vi "Configure Sweep (Step).vi"(0 "VISA resource name":refnum<visa-resource-name>, 1 "Step Spacing (0: Linear)":u16(ring) items=["Linear", "Logarithmic"], 2 "Number Of Points (2)":i32=2, 5 "Step Dwell (2 ms)":dbl=0.002, 7 "Frequency Start (100 kHz)":dbl=100000.0, 9 "Frequency Stop (100 kHz)":dbl=100000.0, 11 "error in (no error)":errorcluster, 12 "Power Start (-130 dB)":dbl=-130.0, 13 "Power Stop (-130 dB)":dbl=-130.0) -> (4 "VISA resource name out":refnum<visa-resource-name>, 15 "error out":errorcluster)   [LabVIEW 2009, in "Agilent PSG MXG Series.lvlib"]
doc: "Configures number of points, dwell time, start frequency, stop frequency, start amplitude and stop amplitude in the step sweep mode."
uses:
  Agilent PSG MXG Series.lvlib
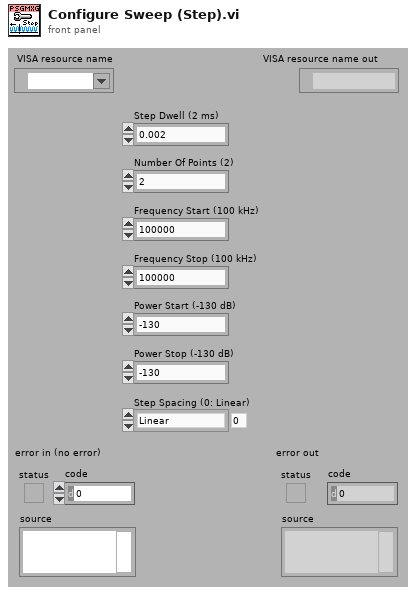
[diagram p1: front panel]
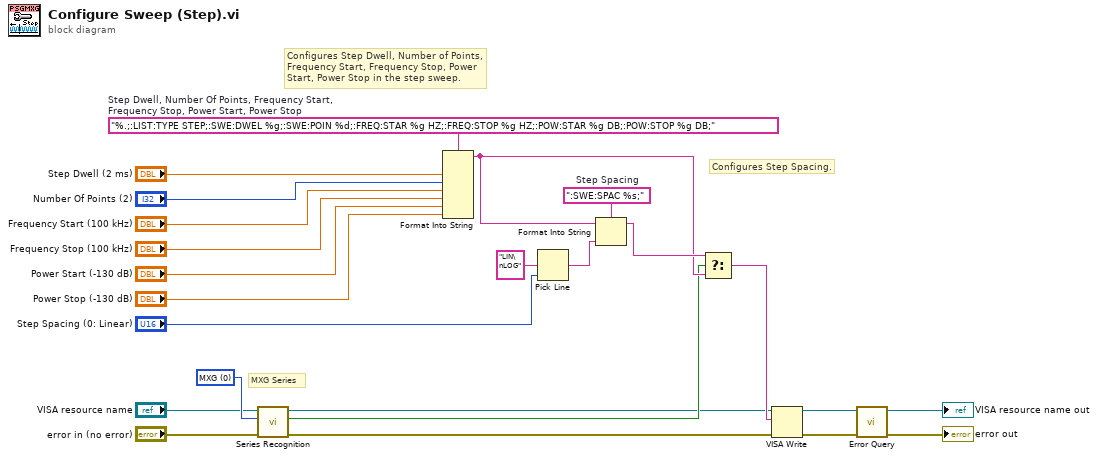
[diagram p0: block diagram]
diagram:
  w5 = u16 0 items=["MXG", "PSG", "PSG-A", "PSG-C", "PSG-D"] ("Series Type (0: MXG)")
  w17 = ":SWE:SPAC %s;"  # Step Spacing
  w24 = "%.;:LIST:TYPE STEP;:SWE:DWEL %g;:SWE:POIN %d;:FREQ:STAR %g HZ;:FREQ:STOP %g HZ;:POW:STAR %g DB;:POW:STOP %g DB;"  # Step Dwell, Number Of Points, Frequency Start, Frequency Stop, Power Start, Power Stop
  # "MXG Series"
  # "Configures Step Spacing."
  # "Configures Step Dwell, Number of Points,\nFrequency Start, Frequency Stop, Power\nStart, Power Stop in the step sweep."
  n1 = call "Series Recognition.vi"("error in (no error)"="error in (no error)", "Series Type (0: MXG)"=w5, "VISA resource name"="VISA resource name") -> ("error out"=w6:errorcluster, "Is Series Correct"=w8:bool, "VISA resource name out"=w7:refnum<visa-resource-name>)  [unwired: 1 in, 5 out]
  n2 = Format Into String(format string=w24, "Step Dwell (2 ms)", "Number Of Points (2)", "Frequency Start (100 kHz)", "Frequency Stop (100 kHz)", "Power Start (-130 dB)", "Power Stop (-130 dB)") -> (resulting string=w12:string)  [unwired: 2 in, 1 out]
  n3 = Pick Line(multi-line string="LIN\nLOG", line index="Step Spacing (0: Linear)") -> (output string=w16:string)  [unwired: 1 out]
  n4 = Format Into String(format string=w17, initial string=w12, w16) -> (resulting string=w13:string)  [unwired: 1 in, 1 out]
  n5 = Select(t=w13, s=w8, f=w12) -> (s? t:f=w11:string)
  n6 = VISA Write(VISA resource name=w7, write buffer=w11, error in (no error)=w6) -> (VISA resource name out=w10:refnum<visa-resource-name>, error out=w9:errorcluster)  [unwired: 1 out]
  n7 = call "Error Query.vi"("error in (no error)"=w9, "VISA resource name"=w10) -> ("error out"=→"error out":errorcluster, "VISA resource name out"=→"VISA resource name out":refnum<visa-resource-name>)  [unwired: 8 out]
